vi "Function_Find Edge #.vi"(8 "Error in":errorcluster, 9 "CoordSys In":T1 {"Measurement System"."Axis Reference" items=["Direct", "Indirect"]; "Measurement System"."Angle (deg)" format="%.2f"; "Measurement System"."Origin"."Y" format="%.2f"; "Measurement System"."Origin"."X" format="%.2f"; "Reference System"."Axis Reference" items=["Direct", "Indirect"]; "Reference System"."Angle (deg)" format="%.2f"; "Reference System"."Origin"."Y" format="%.2f"; "Reference System"."Origin"."X" format="%.2f"}, 10 "Data Cluster In":cluster{"Name":string, "Variant In":variant}, 11 "Image Src":T3) -> (0 "Error Out":errorcluster, 1 "Perpendicular Line(Offset)":T2, 2 "Fit Line(Offset)":T2, 3 "Result":cluster{"Name":string, "NG?":bool, "Score":dbl}, 4 "Time":u32)   [LabVIEW 2013]
uses:
  <vilib>/vision/Image Controls.llb/IMAQ Image.ctl
  Control/Control Find Edge #.ctl
  <vilib>/vision/Measure.llb/Edge Options.ctl
  <vilib>/vision/Measure.llb/Edge Polarity.ctl
  <vilib>/vision/NI_Vision_Development_Module.lvlib
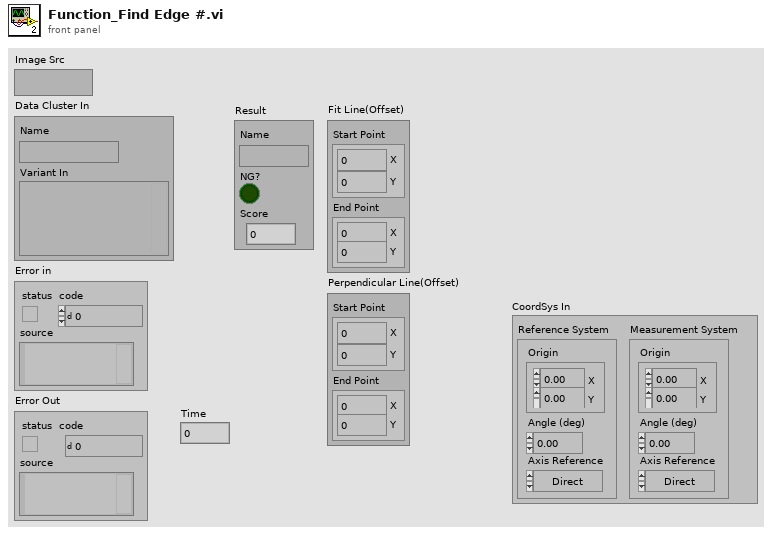
[diagram p1: front panel]
types:
  T1 = typedef "IMAQ Coordinate System" = cluster{"Reference System":cluster{"Origin":cluster{"X":sgl, "Y":sgl}, "Angle (deg)":sgl, "Axis Reference":u32}, "Measurement System":cluster{"Origin":cluster{"X":sgl, "Y":sgl}, "Angle (deg)":sgl, "Axis Reference":u32}}
  T2 = cluster{"Start Point":cluster{"X":i32, "Y":i32}, "End Point":cluster{"X":i32, "Y":i32}}
  T3 = typedef "IMAQ Image.ctl" = refnum<image>
  T4 = typedef "Control Find Edge #.ctl" = cluster{"ROI Descriptor":cluster{"Global Rectangle":i32[], "Contours":cluster{"ID":enum32{"External", "Internal"}, "Type":u32, "Coordinates":i32[]}[]}, "Edge Options":cluster{"Edge Options":T5, "Scan Direction":u16, "Step Size":u32, "SD":dbl, "Auto":bool}, "條件(Line)":cluster{"毛邊長度":dbl}}
  T5 = typedef "Edge Options.ctl" = cluster{"Edge Polarity":T6, "Kernel Size":u32, "Width":u32, "Minimum Edge Strength":sgl, "Interpolation Type":enum32{"Zero Order", "Bilinear", "Quadratic", "Cubic", "Bilinear Fixed"}, "Data Processing Method":enum32{"Average", "Median"}}
  T6 = typedef "Edge Polarity.ctl" = u32
  T7 = cluster{"Global Rectangle":i32[], "Contours":cluster{"ID":enum32{"External", "Internal"}, "Type":u32, "Coordinates":i32[]}[]}
  T8 = cluster{"Origin":cluster{"X":sgl, "Y":sgl}, "Angle (deg)":sgl, "Axis Reference":u32}
  T9 = typedef "ROI Descriptor" = cluster{"Global Rectangle":i32[], "Contours":cluster{"ID":enum32{"External", "Internal"}, "Type":u32, "Coordinates":i32[]}[]}
  T10 = cluster{"Point 1":cluster{"X":i32, "Y":i32}, "Point 2":cluster{"X":i32, "Y":i32}}
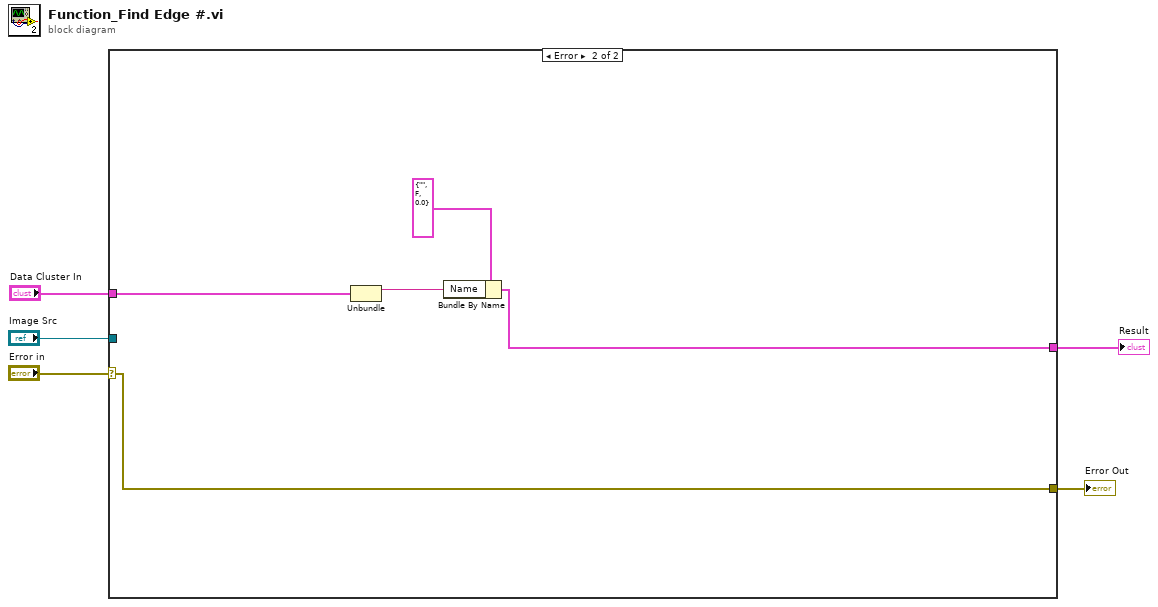
[diagram p0: block diagram]
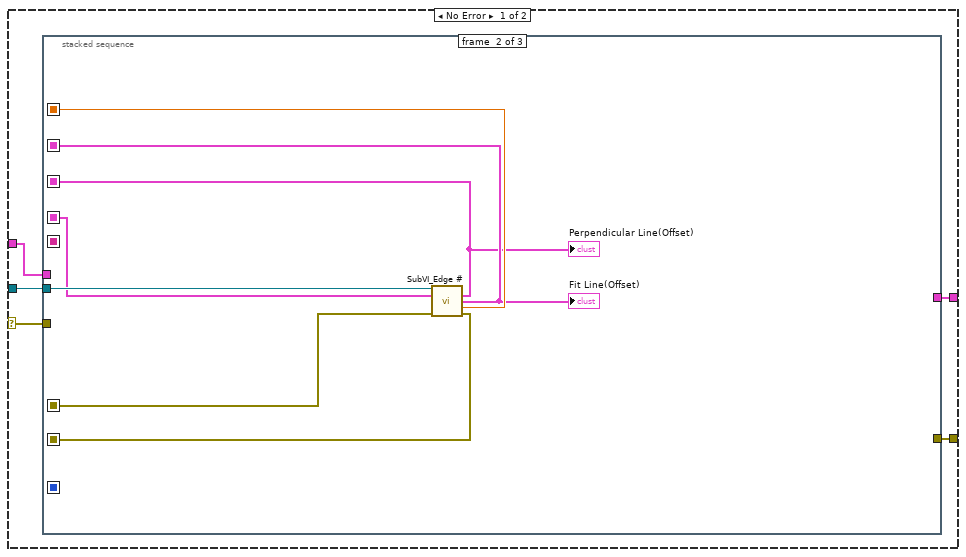
[diagram p2: hidden frame]
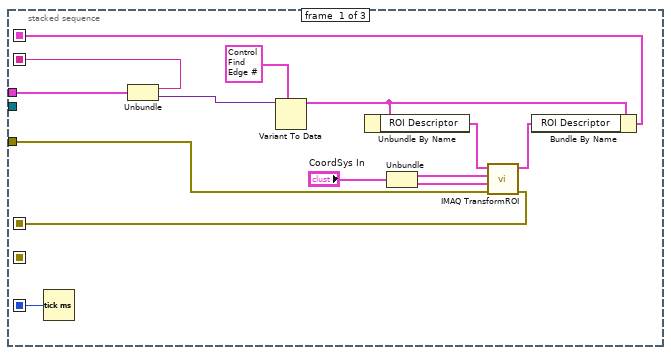
[diagram p3: hidden frame]
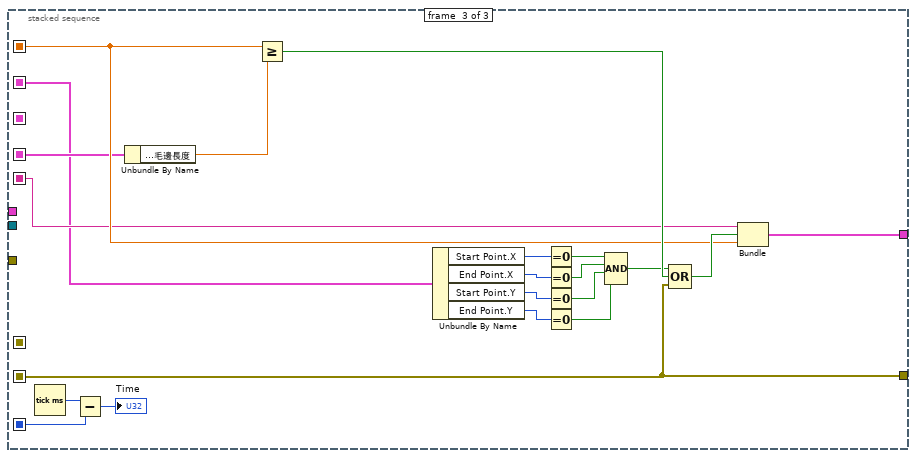
[diagram p4: hidden frame]
diagram:
  n1 = case shown="Error" "Error in" {
    selector: "Error in" -> [w8 w57]
    tunnel: "Image Src" -> [w10 _]
    tunnel: [w9 w57] -> w4
    tunnel: [w7 w53] -> w2
    tunnel: "Data Cluster In" -> [w6 w54]
    frame No Error {
      n2 = stacked-sequence {
        seq-local: [w16 _ _] -> [_ w28 w45]
        seq-local: [w23 _ _] -> [_ _ w51]
        seq-local: [_ w26 _] -> [_ _ _]
        seq-local: [_ w27 _] -> [_ _ w34]
        seq-local: [_ w30 _] -> [_ _ w46]
        seq-local: [_ w29 _] -> [_ _ w44]
        seq-local: [w21 _ _] -> [_ _ w43]
        seq-local: [w12 _ _] -> [_ w25 _]
        tunnel: w8 -> [w13 _ _]
        tunnel: w10 -> [_ w31 _]
        tunnel: [_ _ w44] -> w9
        tunnel: [_ _ w32] -> w7
        tunnel: w6 -> [w11 _ _]
        frame #0 {
          n3 = Tick Count (ms)() -> (millisecond timer value=w23:u32)
          n4 = Unbundle(w11) -> ("Name"=w21:string, "Variant In"=w24:variant)
          n5 = Variant To Data(type=T4 {"ROI Descriptor"={"Global Rectangle"=[], "Contours"=[]}, "Edge Options"={"Edge Options"={"Edge Polarity"=0, "Kernel Size"=0, "Width"=0, "Minimum Edge Strength"=0.0, "Interpolation Type"=enum."Zero Order", "Data Processing Method"=enum."Average"}, "Scan Direction"=0, "Step Size"=0, "SD"=0.0, "Auto"=FALSE}, "條件(Line)"={"毛邊長度"=0.0}} ("Parameter_Edge"), Variant=w24) -> (data=w15:T4)  [unwired: 1 in, 1 out]
          n6 = Unbundle By Name(w15) -> ("ROI Descriptor"=w17:T7)
          n7 = Unbundle("CoordSys In") -> ("Reference System"=w19:T8, "Measurement System"=w20:T8)
          n8 = call "IMAQ TransformROI"("error in (no error)"=w13, "New Reference"=w20, "Base Reference"=w19, "ROI Descriptor"=w17) -> ("error out"=w12:errorcluster, "ROI Descriptor out"=w14:T9)  [unwired: 6 in]
          n9 = Bundle By Name(cluster=w15, "ROI Descriptor"=w14) -> (w16:T4)
        }
        frame #1 {
          n10 = call "SubVI_Edge #.vi"("Image in"=w31, "Parameter_Edge"=w28, "error in"=w25) -> ("Perpendicular Line"=w26:T10, "Fit Line"=w27:T2, "Distance"=w30:dbl, "error out"=w29:errorcluster)  [unwired: 8 in, 1 out]
          "Perpendicular Line(Offset)" <- w26
          "Fit Line(Offset)" <- w27
        }
        frame #2 {
          n11 = Tick Count (ms)() -> (millisecond timer value=w52:u32)
          n12 = Subtract(x=w52, y=w51) -> (x-y=→"Time":u32)
          n13 = Unbundle By Name(w45) -> ("條件(Line).毛邊長度"=w47:dbl)
          n14 = Greater Or Equal?(x=w46, y=w47) -> (x >= y?=w48:bool)
          n15 = Unbundle By Name(w34) -> ("Start Point.X"=w35:i32, "End Point.X"=w36:i32, "Start Point.Y"=w37:i32, "End Point.Y"=w38:i32)
          n16 = Equal To 0?(x=w35) -> (x = 0?=w39:bool)
          n17 = Equal To 0?(x=w36) -> (x = 0?=w40:bool)
          n18 = Equal To 0?(x=w37) -> (x = 0?=w41:bool)
          n19 = Equal To 0?(x=w38) -> (x = 0?=w42:bool)
          n20 = Compound Arithmetic op=AND(w39, w40, w41, w42) -> (w33:bool)
          n21 = Compound Arithmetic op=OR(w33, w48, w44) -> (w49:bool)
          n22 = Bundle("Name"=w43, w49, "Distance"=w46) -> (w32:cluster{"Name":string, bool, "Distance":dbl})  [unwired: 1 in]
        }
      }
    }
    frame Error {
      n23 = Unbundle(w54) -> ("Name"=w55:string)  [unwired: 1 out]
      n24 = Bundle By Name(cluster=cluster{"Name":string, bool, "Radius":dbl} {"Name"="", FALSE, "Radius"=0.0}, "Name"=w55) -> (w53:cluster{"Name":string, bool, "Radius":dbl})
    }
  }
  "Error Out" <- w4
  "Result" <- w2
